vi "Push.vi"(8 "error in (no error)":errorcluster, 10 "Element":dbl, 11 "Stack in":refnum<class "Stack.lvclass">) -> (0 "error out":errorcluster, 3 "Stack out":refnum<class "Stack.lvclass">)   [LabVIEW 2012, in "Stack.lvlib" / "Stack.lvclass"]
doc: "Push an element on top of stack."
uses:
  Stack.lvclass
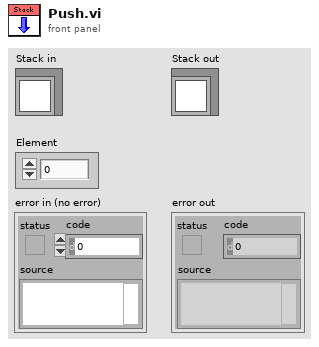
[diagram p1: front panel]
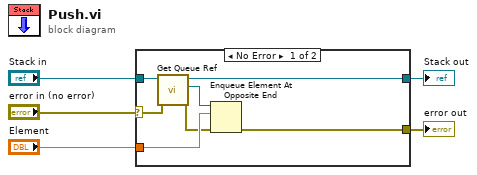
[diagram p0: block diagram]
diagram:
  n1 = case shown="No Error" "error in (no error)" {
    selector: "error in (no error)" -> [w7 w14]
    tunnel: [w6 w14] -> w4
    tunnel: [w11 w13] -> w2
    tunnel: "Stack in" -> [w12 w13]
    tunnel: "Element" -> [w9 _]
    frame No Error {
      n2 = call "Get Queue Ref.vi"("error in (no error)"=w7, "Stack in"=w12) -> ("error out"=w8:errorcluster, "queue out"=w10:refnum<queue>, "Stack out"=w11:refnum<class "Stack.lvclass">)  [unwired: 7 in]
      n3 = Enqueue Element At Opposite End(queue=w10, element=w9, error in (no error)=w8) -> (error out=w6:errorcluster)  [unwired: 1 in, 2 out]
    }
    frame Error {
    }
  }
  "error out" <- w4
  "Stack out" <- w2
